vi "Pose2d_Times.vi"(9 "Scalar":dbl, 11 "in POSE":T1 {"ROTATION"."SIN" format="%13.4f"; "ROTATION"."COS" format="%13.4f"; "ROTATION"."VALUE" format="%13.4f"; "TRANSLATION"."Y" format="%14.3f"; "TRANSLATION"."X" format="%14.3f"}) -> (3 "out POSE":T1 {"ROTATION"."SIN" format="%13.4f"; "ROTATION"."COS" format="%13.4f"; "ROTATION"."VALUE" format="%13.4f"; "TRANSLATION"."Y" format="%14.3f"; "TRANSLATION"."X" format="%14.3f"})   [LabVIEW 2019, in "Trajectory_Library.lvlib"]
doc: "Multiply the pose by the given scalar\"\n\n\nParameters:\n - IN POSE - The input POSE data structure\n - Scalar - The value to multiply the pose by.\n\nReturn:\n - OUT POSE - The output pose."
uses:
  TypeDef/POSE2D.ctl
  TypeDef/TRANSLATION2D.ctl
  TypeDef/ROTATION2D.ctl
  Translation2d_RotateBy.vi
  Translation2d_Plus.vi
  Rotation2d_Plus.vi
  Rotation2d_RotateBy.vi
  Rotation2d_CreateXY.vi
  Util_CalcDist.vi
  Trajectory_Library.lvlib
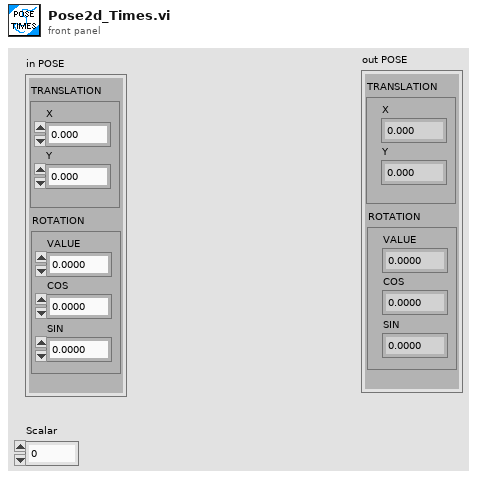
[diagram p1: front panel]
types:
  T1 = typedef "Trajectory_Library.lvlib/POSE2D.ctl" = cluster{"TRANSLATION":T2, "ROTATION":T3}
  T2 = typedef "Trajectory_Library.lvlib/TRANSLATION2D.ctl" = cluster{"X":dbl, "Y":dbl}
  T3 = typedef "Trajectory_Library.lvlib/ROTATION2D.ctl" = cluster{"VALUE":dbl, "COS":dbl, "SIN":dbl}
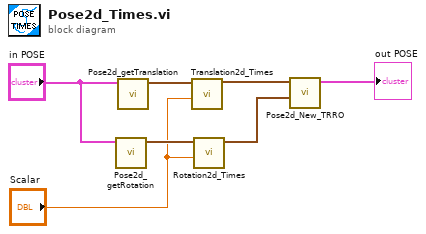
[diagram p0: block diagram]
diagram:
  n1 = call "Pose2d_getRotation.vi"("in POSE"="in POSE") -> ("out ROTATION"=w5:T3)  [unwired: 10 in]
  n2 = call "Pose2d_getTranslation.vi"("in POSE"="in POSE") -> ("outTRANSLATION"=w6:T2)  [unwired: 10 in]
  n3 = call "Translation2d_Times.vi"("Scalar"="Scalar", "In Translation"=w6) -> ("Out Translation"=w3:T2)  [unwired: 9 in]
  n4 = call "Rotation2d_Times.vi"("Scalar"="Scalar", "in ROTATION"=w5) -> ("out ROTATION"=w2:T3)  [unwired: 9 in]
  n5 = call "Pose2d_New_TRRO.vi"("ROTATION"=w2, "TRANSLATION"=w3) -> ("outPOSE"=→"out POSE":T1)  [unwired: 9 in]
